vi "Actor Core.vi"(8 "error in":errorcluster, 11 "CommonState in":refnum<class "CoordinatorState.lvclass">) -> (0 "error out":errorcluster, 3 "Actor out":refnum<class "Actor.lvclass">)   [LabVIEW 2014, in "States.lvlib" / "CoordinatorState.lvclass"]
doc: "(<B>Filename</B>: Actor Framework.lvlib:Actor.lvclass:Actor Core.vi)\n\n\nThis override launches an instance of Process Actor.lvclass.\n\nReceives messages to the actor, reacts to them, and initiates any error handling that may shut the actor down.\n\nDescendant classes may override this VI to append parallel tasks for the actor to complete while it handles messages. Overrides use the Call Parent Method node."
uses:
  CoordinatorState.lvclass
  <vilib>/ActorFramework/Actor/Actor.lvclass
  Map_lib/MapBuilder/Robot_Position.ctl
  ControlPanel_lib/Input Operator/ControlPanel.lvclass
  Map_lib/MapDisplayer/Map.lvclass
  RemoteP3AT_lib/Remote P3AT/RemoteP3AT.lvclass
  GlobalPlannerPyPl/GlobalPlannerPyPlActor/GlobalPlannerPyPl.lvclass
  <vilib>/ActorFramework/Actor/Actor.lvclass/Actor.ctl
  <vilib>/ActorFramework/Message Enqueuer/Message Enqueuer.lvclass/Message Enqueuer.ctl
  CoordinatorState.lvclass/CoordinatorState.ctl
  <vilib>/ActorFramework/Message Enqueuer/Enqueue.vi
  <vilib>/ActorFramework/Message Enqueuer/Init from Existing Queue.vi
  <vilib>/ActorFramework/Message Priority Queue/Priority Enqueue.vi
  <vilib>/ActorFramework/Message Enqueuer/Message Enqueuer.lvclass
  GlobalPlanner_lib/GlobalPlanner/GlobalPlanner.lvclass
  <vilib>/NI/Actors/State Actor/State Actor/State Actor.lvclass
panel:
  out "vel_cal":cluster{"rot_z":dbl, "lin_x":dbl}
  out "MapPosition":T1
  out "P3AT_Ini_Pose":T2
  out "robot position":T3
  out "sensor":cluster{"voltage":dbl, "motor":i8}
  in  "停止信号":bool
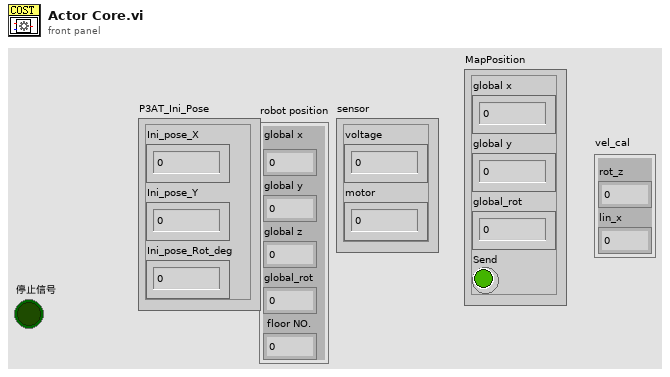
[diagram p1: front panel]
types:
  T1 = cluster{"global x":dbl, "global y":dbl, "global_rot":dbl, "Send":bool}
  T2 = cluster{"Ini_pose_X":dbl, "Ini_pose_Y":dbl, "Ini_pose_Rot_deg":dbl}
  T3 = typedef "Robot_Position.ctl" = cluster{"global x":dbl, "global y":dbl, "global z":dbl, "global_rot":dbl, " floor NO.":dbl}
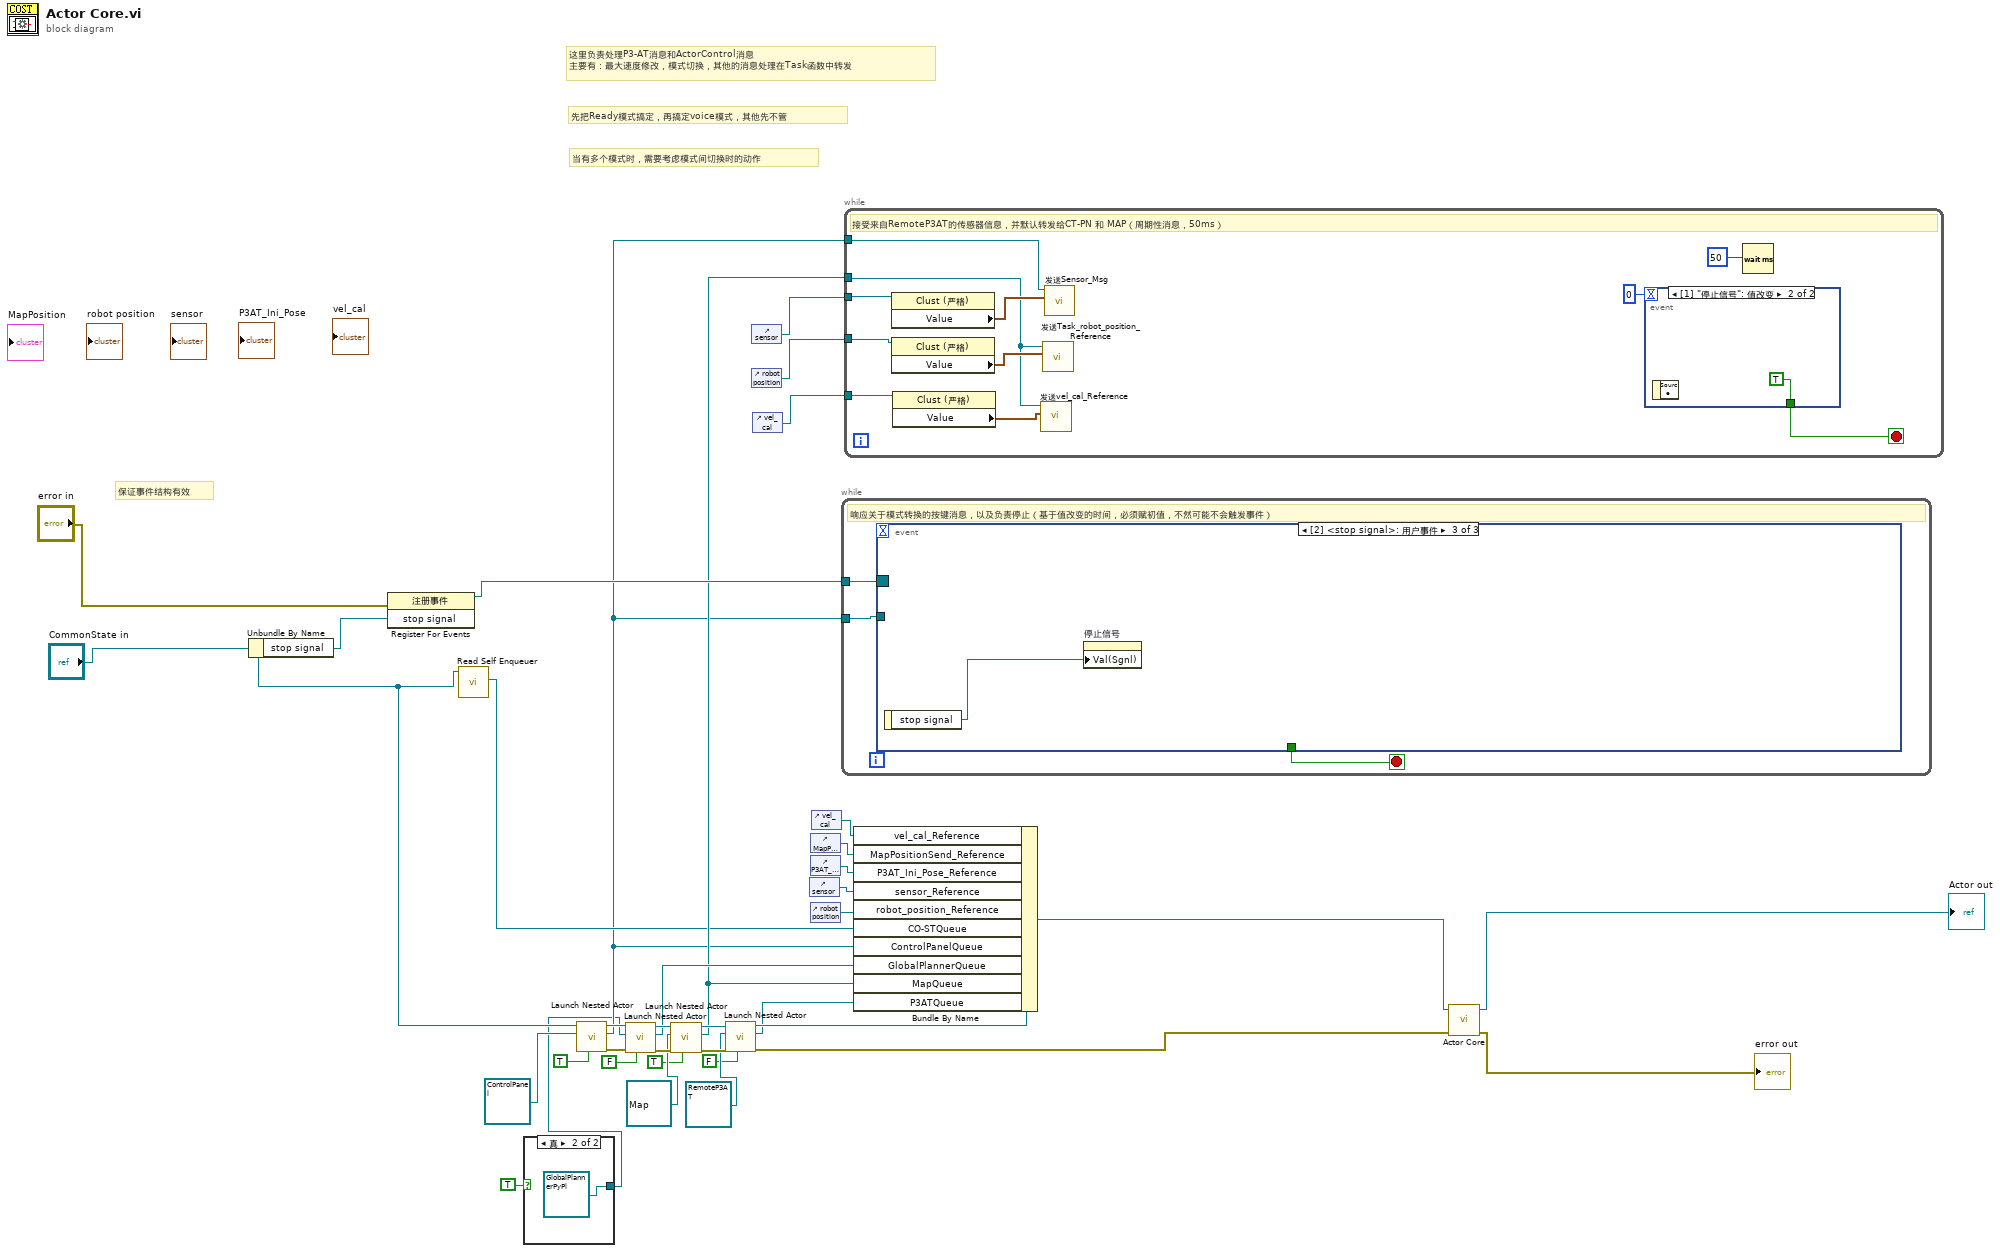
[diagram p0: block diagram]
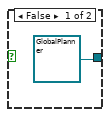
[diagram p2: hidden frame]
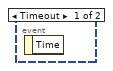
[diagram p3: hidden frame]
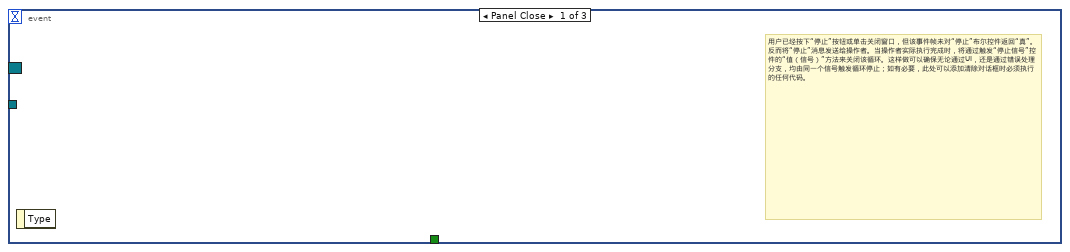
[diagram p4: hidden frame]
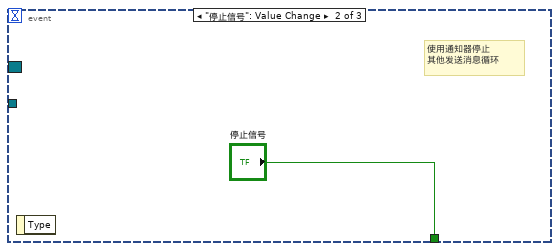
[diagram p5: hidden frame]
diagram:
  # "保证事件结构有效"
  # "当有多个模式时，需要考虑模式间切换时的动作"
  # "先把Ready模式搞定，再搞定voice模式，其他先不管"
  # "这里负责处理P3-AT消息和ActorControl消息\n主要有：最大速度修改，模式切换，其他的消息处理在Task函数中转发"
  n1 = Unbundle By Name("CommonState in") -> ("stop signal"=w17:refnum<user-event>)
  n2 = register-events(error in="error in", w17) -> (reference out=w19:refnum<event-registration>)  [unwired: 1 in, 1 out]
  n3 = call <vilib>:"Read Self Enqueuer.vi"("Actor"="CommonState in") -> ("Self Enqueuer"=w16:refnum<class "Message Enqueuer.lvclass">)  [unwired: 10 in]
  n4 = case shown="真" TRUE {
    tunnel: [refnum<class "GlobalPlanner.lvclass"> refnum ("GlobalPlanner.lvlib:GlobalPlanner.lvclass") refnum<class "GlobalPlannerPyPl.lvclass"> refnum ("GlobalPlannerPyPl.lvlib:GlobalPlannerPyPl.lvclass")] -> w1
    frame False {
    }
    frame True {
    }
  }
  n5 = call <vilib>:"Launch Nested Actor.vi"("Open Actor Core front panel? (F)"=TRUE, "Nested Actor"=refnum<class "ControlPanel.lvclass"> refnum ("ControlPanel.lvlib:ControlPanel.lvclass"), "Caller Actor in"="CommonState in") -> ("error out"=w29:errorcluster, "Nested Actor's Enqueuer"=w9:refnum<class "Message Enqueuer.lvclass">, "Caller Actor out"=w28:refnum<class "CoordinatorState.lvclass">)  [unwired: 6 in]
  n6 = call <vilib>:"Launch Nested Actor.vi"("Open Actor Core front panel? (F)"=FALSE, "error in (no error)"=w29, "Nested Actor"=w1, "Caller Actor in"=w28) -> ("error out"=w31:errorcluster, "Nested Actor's Enqueuer"=w25:refnum<class "Message Enqueuer.lvclass">, "Caller Actor out"=w30:refnum<class "CoordinatorState.lvclass">)  [unwired: 5 in]
  n7 = call <vilib>:"Launch Nested Actor.vi"("Open Actor Core front panel? (F)"=TRUE, "error in (no error)"=w31, "Nested Actor"=refnum<class "Map.lvclass"> refnum ("Map.lvlib:Map.lvclass"), "Caller Actor in"=w30) -> ("error out"=w33:errorcluster, "Nested Actor's Enqueuer"=w18:refnum<class "Message Enqueuer.lvclass">, "Caller Actor out"=w32:refnum<class "CoordinatorState.lvclass">)  [unwired: 5 in]
  n8 = call <vilib>:"Launch Nested Actor.vi"("Open Actor Core front panel? (F)"=FALSE, "error in (no error)"=w33, "Nested Actor"=refnum<class "RemoteP3AT.lvclass"> refnum ("RemoteP3AT.lvlib:RemoteP3AT.lvclass"), "Caller Actor in"=w32) -> ("error out"=w34:errorcluster, "Nested Actor's Enqueuer"=w23:refnum<class "Message Enqueuer.lvclass">, "Caller Actor out"=w24:refnum<class "CoordinatorState.lvclass">)  [unwired: 5 in]
  n9 = control-ref of="sensor"() -> (w13:refnum<vi>)
  n10 = control-ref of="robot position"() -> (w12:refnum<vi>)
  n11 = control-ref of="vel_cal"() -> (w3:refnum<vi>)
  n12 = control-ref of="sensor"() -> (w15:refnum<vi>)
  n13 = control-ref of="MapPosition"() -> (w5:refnum<vi>)
  n14 = control-ref of="P3AT_Ini_Pose"() -> (w11:refnum<vi>)
  n15 = control-ref of="robot position"() -> (w14:refnum<vi>)
  n16 = control-ref of="vel_cal"() -> (w4:refnum<vi>)
  n17 = while {
    tunnel: w19 -> [w41]
    tunnel: w9 -> [w40]
    stop <- w42 stop-if-true
    # "响应关于模式转换的按键消息，以及负责停止（基于值改变的时间，必须赋初值，不然可能不会触发事件）"
    n18 = event shown="[2] <stop signal>: 用户事件" {
      selector: w41 -> [_ _ _]
      dyn-events: _ -> [_ _ _]
      timeout: _ -> [_ _ _]
      tunnel: [_ "停止信号" _] -> w42
      tunnel: w40 -> [_ _ _]
      event Panel Close {
        # "用户已经按下“停止”按钮或单击关闭窗口，但该事件帧未对“停止”布尔控件返回“真”。反而将“停止”消息发送给操作者。当操作者实际执行完成时，将通过触发“停止信号”控件的“值（信号）”方法来关闭该循环。这样做可以确保无论通过UI，还是通过错误处理分支，均由同一个信号触发循环停止；如有必要，此处可以添加清除对话框时必须执行的任何代码。"
        n19 = event-data() -> ()  [unwired: 1 in, 1 out]
      }
      event "停止信号": Value Change {
        # "使用通知器停止\n其他发送消息循环"
        n20 = event-data() -> ()  [unwired: 1 in, 1 out]
      }
      event User Event {
        n21 = event-data() -> ("stop signal"=w44:bool)  [unwired: 1 in]
        n22 = property on="停止信号" class="Bool (严格)"("Val(Sgnl)"=w44) -> ()  [unwired: 2 in, 2 out]
      }
    }
  }
  n23 = while {
    tunnel: w9 -> [w50]
    tunnel: w18 -> [w46]
    tunnel: w13 -> [w52]
    tunnel: w12 -> [w51]
    tunnel: w3 -> [w47]
    stop <- w53 stop-if-true
    # "接受来自RemoteP3AT的传感器信息，并默认转发给CT-PN 和 MAP（周期性消息，50ms）"
    n24 = property class="Clust (严格)"(reference=w52) -> ("Value"=w49:cluster{"voltage":dbl, "motor":i8})  [unwired: 1 in, 2 out]
    n25 = property class="Clust (严格)"(reference=w51) -> ("Value"=w48:T3)  [unwired: 1 in, 2 out]
    n26 = property class="Clust (严格)"(reference=w47) -> ("Value"=w45:cluster{"rot_z":dbl, "lin_x":dbl})  [unwired: 1 in, 2 out]
    n27 = call "发送vel_cal_Reference.vi"("值(信号)"=w45, "消息待入队列"=w46) -> ()  [unwired: 8 in, 2 out]
    n28 = call "发送Task_robot_position_Reference.vi"("值(信号)"=w48, "消息待入队列"=w46) -> ()  [unwired: 8 in, 2 out]
    n29 = call "发送Sensor_Msg.vi"("sensor"=w49, "消息待入队列"=w50) -> ()  [unwired: 8 in, 2 out]
    n30 = event shown="[1] \"停止信号\": 值改变" {
      selector: _ -> [_ _]
      dyn-events: _ -> [_ _]
      timeout: 0 -> [_ _]
      tunnel: [_ TRUE] -> w53
      event Timeout {
        n31 = event-data() -> ()  [unwired: 1 in, 1 out]
      }
      event "停止信号": Value Change {
        n32 = event-data() -> ()  [unwired: 1 in, 1 out]
      }
    }
    n33 = Wait (ms)(milliseconds to wait=u32 50 ("等待时间（毫秒）")) -> ()  [unwired: 1 out]
  }
  n34 = Bundle By Name(cluster=w24, "vel_cal_Reference"=w4, "MapPositionSend_Reference"=w5, "P3AT_Ini_Pose_Reference"=w11, "sensor_Reference"=w15, "robot_position_Reference"=w14, "CO-STQueue"=w16, "ControlPanelQueue"=w9, "GlobalPlannerQueue"=w25, "MapQueue"=w18, "P3ATQueue"=w23) -> (w36:refnum<class "CoordinatorState.lvclass">)
  n35 = call-parent "Actor Core.vi"("error in"=w34, "State in"=w36) -> ("error out"=→"error out":errorcluster, "Actor out"=→"Actor out":refnum<class "Actor.lvclass">)  [unwired: 8 in]
